vi "rtin_ControlNslMux.vi"(7 "Set":bool, 8 "error in":errorcluster, 10 "axis in":u8, 11 "connection ID":refnum<k5>) -> (0 "error out":errorcluster, 2 "axis out":i32, 3 "connection ID":refnum<k5>)   [LabVIEW 2016]
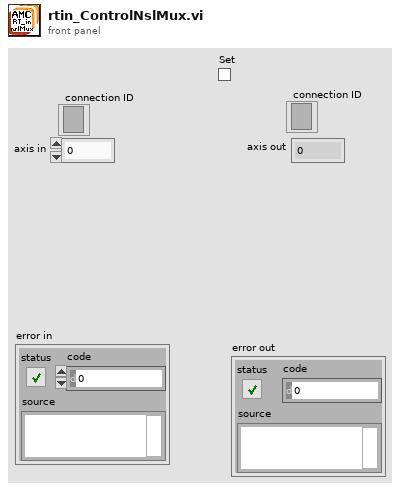
[diagram p1: front panel]
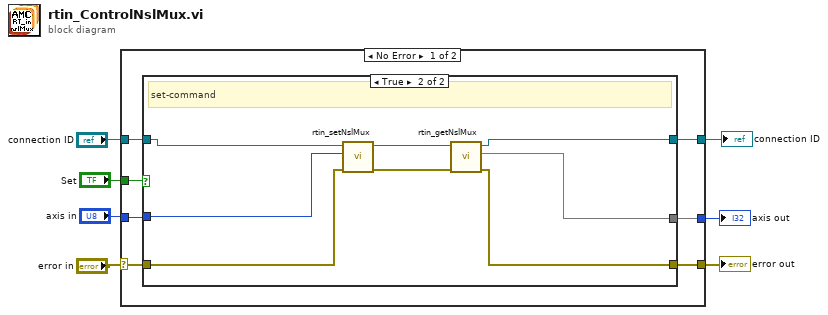
[diagram p0: block diagram]
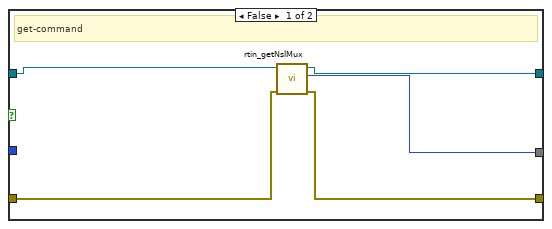
[diagram p2: hidden frame]
diagram:
  n1 = case shown="No Error" "error in" {
    selector: "error in" -> [w11 w30]
    tunnel: "axis in" -> [w14 w28]
    tunnel: [w10 w30] -> w6
    tunnel: "Set" -> [w12 _]
    tunnel: [w9 w29] -> w4
    tunnel: "connection ID" -> [w13 w29]
    tunnel: [w8 w28] -> w1
    frame No Error {
      n2 = case shown="True" w12 {
        tunnel: w13 -> [w19 w22]
        tunnel: w14 -> [_ w21]
        tunnel: w11 -> [w16 w25]
        tunnel: [w17 w24] -> w10
        tunnel: [w18 w23] -> w9
        tunnel: [w15 w20] -> w8
        frame False {
          # "get-command"
          n3 = call "rtin_getNslMux.vi"("error in"=w16, "connection ID"=w19) -> ("error out"=w17:errorcluster, "connection ID"=w18:refnum<k5>, "mux_mode"=w15:i32)  [unwired: 7 in]
        }
        frame True {
          # "set-command"
          n4 = call "rtin_setNslMux.vi"("error in"=w25, "mux_mode"=w21, "connection ID"=w22) -> ("error out"=w27:errorcluster, "connection ID"=w26:refnum<k5>)  [unwired: 7 in]
          n5 = call "rtin_getNslMux.vi"("error in"=w27, "mux_mode"=w20, "connection ID"=w26) -> ("error out"=w24:errorcluster, "connection ID"=w23:refnum<k5>)  [unwired: 7 in]
        }
      }
    }
    frame Error {
    }
  }
  "error out" <- w6
  "axis out" <- w1
  "connection ID" <- w4
